vi "rpm_2_torquesetpoints.vi"(0 "C_d":dbl=0.35, 1 "Density_Air(kg/m^3)":dbl=1.225, 2 "Frontal Area(m^2)":dbl=3.5, 3 "Slope(degrees)":dbl, 4 "Mass(kg)":dbl=1800.0, 7 "Gravitational accelaration(m/s^2)":dbl=9.81, 9 "Rolling Resistance Coefficient C_rf":dbl=0.008, 10 "RPM":dbl, 11 "Tyre Diameter(m)":dbl=0.5) -> (12 "C1":dbl=0.7503125, 13 "C2":dbl=141.264, 14 "D1":dbl=0.00012856402000333957, 15 "Torque Setpoints_graph":dbl, 16 "D2":dbl=35.316, 17 "D3":dbl=11.780972450961723, 19 "C3":dbl=1800.0)   [LabVIEW 2017]
uses:
  <vilib>/ptbypt/NI_PtbyPt.lvlib
panel:
  out "dx/dt":dbl(graph)
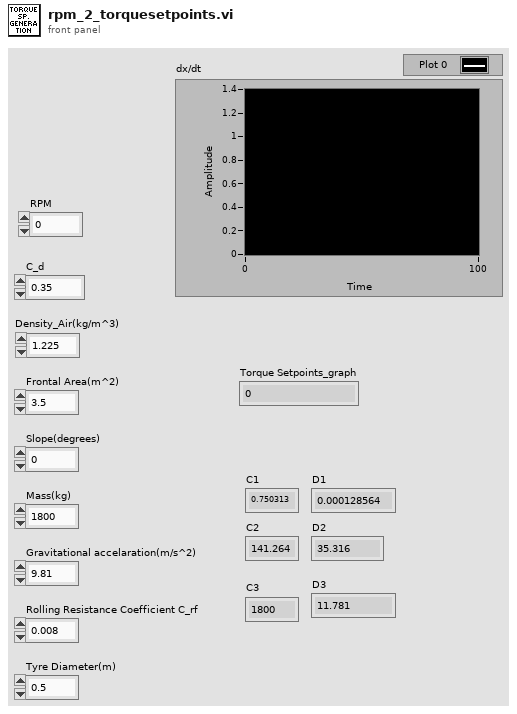
[diagram p1: front panel]
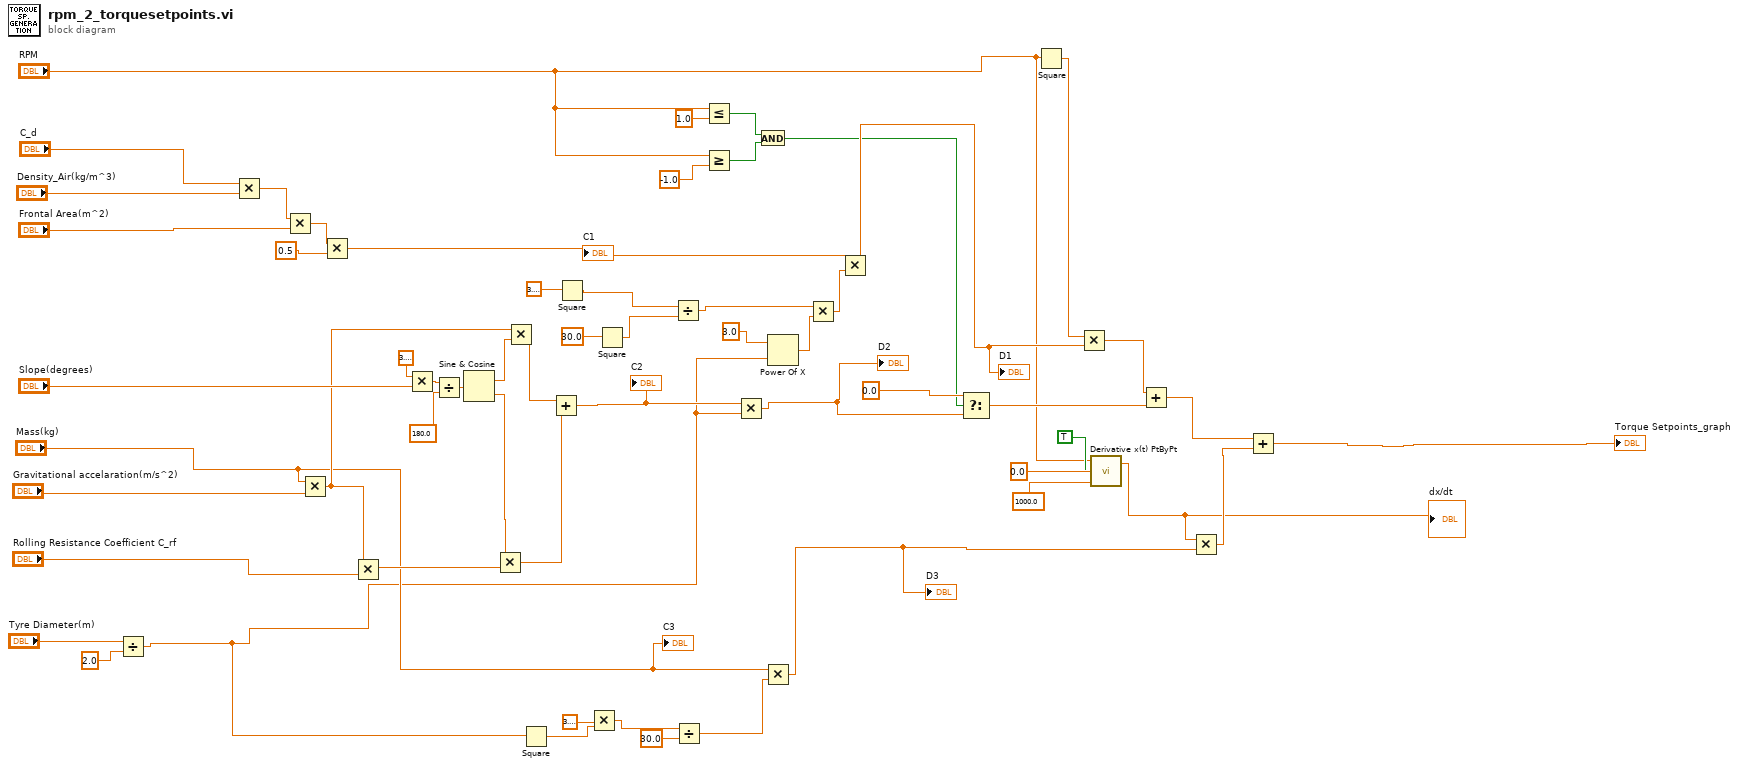
[diagram p0: block diagram]
diagram:
  n1 = Divide(x="Tyre Diameter(m)", y=2.0) -> (x/y=w1:dbl)
  n2 = Multiply(x="C_d", y="Density_Air(kg/m^3)") -> (x*y=w34:dbl)
  n3 = Multiply(x=w34, y="Frontal Area(m^2)") -> (x*y=w36:dbl)
  n4 = Multiply(x="Mass(kg)", y="Gravitational accelaration(m/s^2)") -> (x*y=w42:dbl)
  n5 = Multiply(x=w36, y=0.5 ("x*y")) -> (x*y=w51:dbl)
  "C1" <- w51
  n6 = Multiply(x=w42, y="Rolling Resistance Coefficient C_rf") -> (x*y=w40:dbl)
  n7 = Multiply(x=3.141592653589793, y="Slope(degrees)") -> (x*y=w48:dbl)
  n8 = Divide(x=w48, y=180.0 ("x/y")) -> (x/y=w50:dbl)
  n9 = Sine & Cosine(0:w50) -> (1:w43:dbl, 2:w41:dbl)
  n10 = Multiply(x=w41, y=w40) -> (x*y=w45:dbl)
  n11 = Multiply(x=w42, y=w43) -> (x*y=w44:dbl)
  n12 = Square(x=w1) -> (x^2=w19:dbl)
  n13 = Add(x=w44, y=w45) -> (x+y=w21:dbl)
  "C2" <- w21
  n14 = Square(x=3.141592653589793) -> (x^2=w30:dbl)
  n15 = Multiply(x=3.141592653589793, y=w19) -> (x*y=w18:dbl)
  n16 = Square(x=30.0 ("y")) -> (x^2=w27:dbl)
  n17 = Divide(x=w30, y=w27) -> (x/y=w26:dbl)
  n18 = Divide(x=w18, y=30.0) -> (x/y=w15:dbl)
  n19 = Less Or Equal?(x="RPM", y=1.0) -> (x <= y?=w7:bool)
  n20 = Greater Or Equal?(x="RPM", y=-1.0) -> (x >= y?=w6:bool)
  n21 = Multiply(x=w21, y=w1) -> (x*y=w12:dbl)
  "D2" <- w12
  n22 = And(x=w7, y=w6) -> (x .and. y?=w5:bool)
  n23 = Multiply(x="Mass(kg)", y=w15) -> (x*y=w14:dbl)
  "D3" <- w14
  n24 = Power Of X(1:w1, 2:3.0 ("x^y")) -> (0:w24:dbl)
  n25 = Multiply(x=w26, y=w24) -> (x*y=w25:dbl)
  n26 = Multiply(x=w51, y=w25) -> (x*y=w31:dbl)
  "D1" <- w31
  n27 = Select(t=0.0, s=w5, f=w12) -> (s? t:f=w11:dbl)
  n28 = Square(x="RPM") -> (x^2=w4:dbl)
  n29 = Multiply(x=w4, y=w31) -> (x*y=w52:dbl)
  n30 = call <vilib>:"Derivative x(t) PtByPt.vi"("initialize"=TRUE, "dt"=1000.0, "initial condition"=0.0, "x"="RPM") -> ("dx/dt"=w54:dbl)  [unwired: 1 out]
  "dx/dt" <- w54
  n31 = Add(x=w52, y=w11) -> (x+y=w53:dbl)
  n32 = Multiply(x=w54, y=w14) -> (x*y=w55:dbl)
  n33 = Add(x=w53, y=w55) -> (x+y=→"Torque Setpoints_graph":dbl)
  "C3" <- "Mass(kg)"
